vi "AutoAlignV2.vi"() -> (2 "Wheel":dbl=-0.028555371017094426, 3 "Throttle":dbl=0.03135962260926177)   [LabVIEW 2020]
uses:
  <vilib>/Rock Robotics/Network Tables/NT Read Number.vi
  <vilib>/addons/control/pid/pid.llb/PID (DBL).vi
  <vilib>/addons/control/pid/NI_PID_pid.lvlib
panel:
  in  "multiplication value":dbl=1.0
  in  "OutputRange":cluster{"output high":dbl, "output low":dbl}={"output high"=1.0, "output low"=-1.0} {"output low" format="%.2f"; "output high" format="%.2f"}
  in  "ThrottlePID":T1={"proportional gain (Kc)"=0.018, "integral time (Ti, min)"=0.0, "derivative time (Td, min)"=0.0} {"derivative time (Td, min)" format="%.3f"; "integral time (Ti, min)" format="%.3f"; "proportional gain (Kc)" format="%.3f"}
  in  "WheelPID":T1={"proportional gain (Kc)"=0.006, "integral time (Ti, min)"=0.0, "derivative time (Td, min)"=1e-05} {"derivative time (Td, min)" format="%.9f"; "integral time (Ti, min)" format="%.9f"; "proportional gain (Kc)" format="%.9f"}
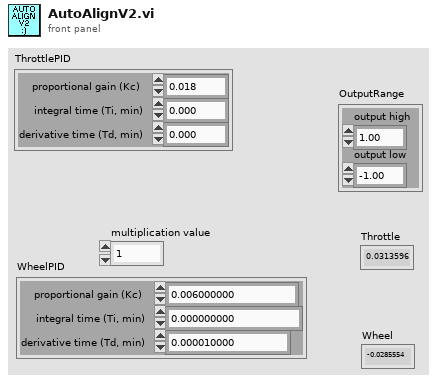
[diagram p1: front panel]
types:
  T1 = cluster{"proportional gain (Kc)":dbl, "integral time (Ti, min)":dbl, "derivative time (Td, min)":dbl}
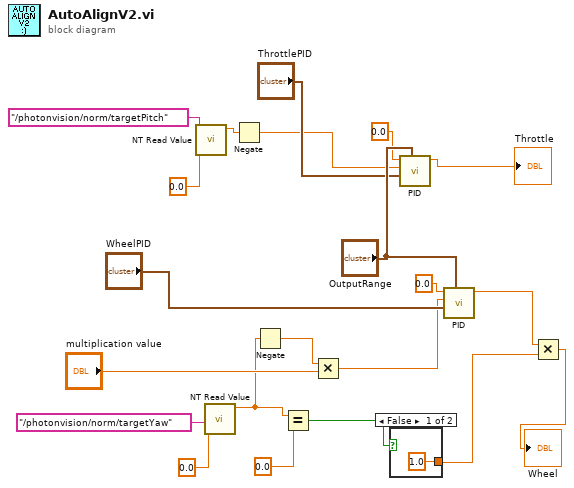
[diagram p0: block diagram]
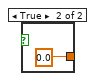
[diagram p2: hidden frame]
diagram:
  n1 = call-poly <vilib>:"NT Read Value.vi"("Default Value"=0.0, "Name"="/photonvision/norm/targetPitch") -> ("Numeric"=w11:dbl)  [unwired: 8 in, 1 out]
  n2 = call-poly <vilib>:"NT Read Value.vi"("Default Value"=0.0, "Name"="/photonvision/norm/targetYaw") -> ("Numeric"=w4:dbl)  [unwired: 8 in, 1 out]
  n3 = Negate(x=w11) -> (-x=w10:dbl)
  n4 = Negate(x=w4) -> (-x=w8:dbl)
  n5 = Equal?(x=w4, y=0.0) -> (x = y?=w2:bool)
  n6 = Multiply(x=w8, y="multiplication value") -> (x*y=w9:dbl)
  n7 = case shown="False" w2 {
    tunnel: [1.0 ("y") 0.0 ("y")] -> w1
    frame False {
    }
    frame True {
    }
  }
  n8 = call-poly <vilib>:"PID.vi"("output range"="OutputRange", "PID gains"="ThrottlePID", "process variable"=w10, "setpoint"=0.0) -> ("output"=→"Throttle":dbl)  [unwired: 6 in, 1 out]
  n9 = call-poly <vilib>:"PID.vi"("output range"="OutputRange", "PID gains"="WheelPID", "process variable"=w9, "setpoint"=0.0) -> ("output"=w6:dbl)  [unwired: 6 in, 1 out]
  n10 = Multiply(x=w6, y=w1) -> (x*y=→"Wheel":dbl)
